vi "3d model.vi"() -> (0 "error out":errorcluster, 1 "Коптер + оси":refnum<vi>, 2 "Вся сцена":refnum<vi>)   [LabVIEW 2013]
uses:
  <vilib>/Utility/miscctls.llb/LV3DPointTypeDef.ctl
  <vilib>/picture/3D Picture Control/Object/Create Object (name).vi
  <vilib>/picture/3D Picture Control/Helpers/Set Light (no reference).vi
  <vilib>/picture/3D Picture Control/NI_3D Picture Control.lvlib
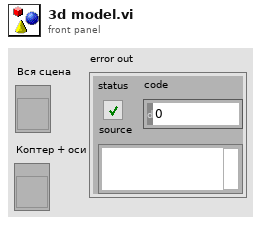
[diagram p1: front panel]
types:
  T1 = cluster{"Red":sgl, "Green":sgl, "Blue":sgl, "Alpha":sgl}
  T2 = typedef "LV3DPointTypeDef.ctl" = cluster{"X":sgl, "Y":sgl, "Z":sgl}
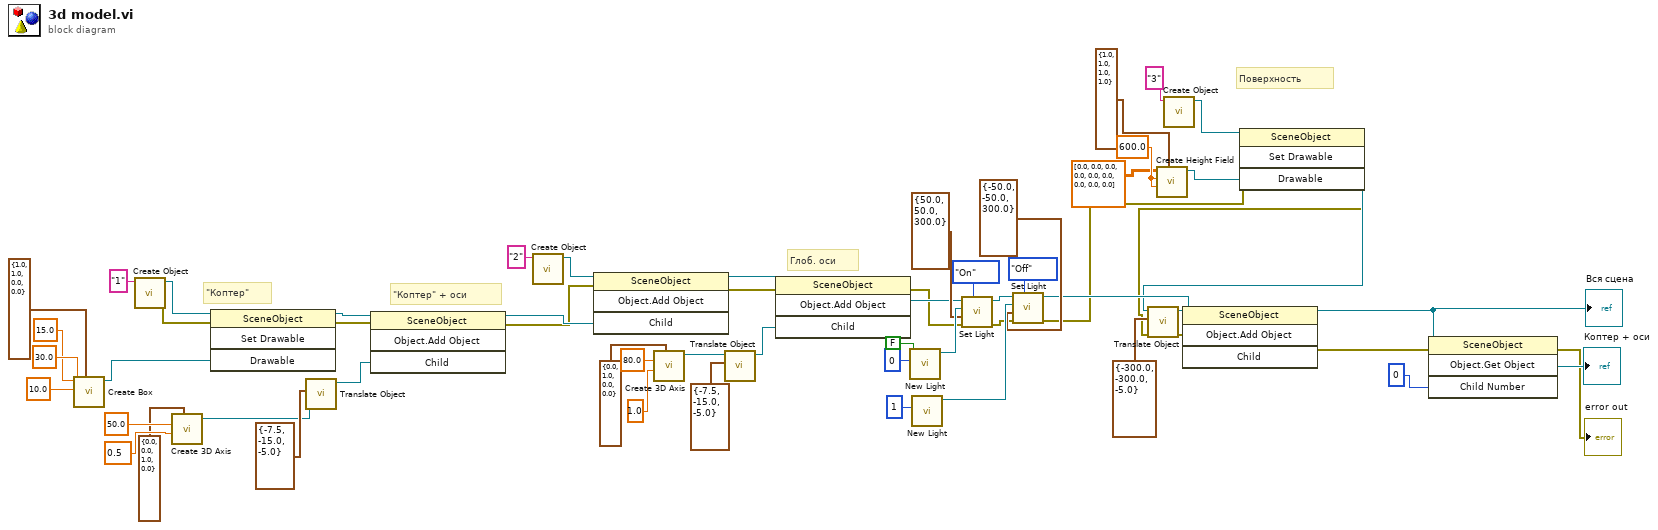
[diagram p0: block diagram]
diagram:
  w44 = sgl 600.0 ("Row Interval")
  # "Глоб. оси"
  # "\"Коптер\" + оси"
  # "\"Коптер\""
  # "Поверхность"
  n1 = call <vilib>:"Create Box.vi"("Color"=T1 {"Red"=1.0, "Green"=1.0, "Blue"=0.0, "Alpha"=0.0}, "Length Z"=sgl 10.0, "Length Y"=sgl 30.0, "Length X"=sgl 15.0) -> ("New Box Refnum"=w15:refnum<vi>)  [unwired: 6 in, 1 out]
  n2 = call-poly <vilib>:"Create Object.vi"("Name"="1") -> ("error out"=w11:errorcluster, "Scene:New Object"=w27:refnum<vi>)  [unwired: 9 in]
  n3 = call <vilib>:"Create 3D Axis.vi"("Color"=T1 {"Red"=0.0, "Green"=0.0, "Blue"=1.0, "Alpha"=0.0}, "Radius"=sgl 0.5, "Length"=sgl 50.0) -> ("New Object Refnum"=w28:refnum<vi>)  [unwired: 7 in, 1 out]
  n4 = invoke class="SceneObject" method="Set Drawable"(reference=w27, error in=w11, "Drawable"=w15) -> (reference out=w33:refnum<vi>, error out=w10:errorcluster)  [unwired: 1 in, 2 out]
  n5 = call <vilib>:"Translate Object.vi"("Translation"=cluster{"X":sgl, "Y":sgl, "Z":sgl} {"X"=-7.5, "Y"=-15.0, "Z"=-5.0}, "Scene.Object In"=w28) -> ("Scene.Object Out"=w34:refnum<vi>)  [unwired: 8 in, 1 out]
  n6 = invoke class="SceneObject" method="Object.Add Object"(reference=w33, error in=w10, "Child"=w34) -> (reference out=w35:refnum<vi>, error out=w9:errorcluster)  [unwired: 1 in, 2 out]
  n7 = call-poly <vilib>:"Create Object.vi"("Name"="2") -> ("Scene:New Object"=w22:refnum<vi>)  [unwired: 9 in, 1 out]
  n8 = invoke class="SceneObject" method="Object.Add Object"(reference=w22, error in=w9, "Child"=w35) -> (reference out=w25:refnum<vi>, error out=w8:errorcluster)  [unwired: 1 in, 2 out]
  n9 = call <vilib>:"Create 3D Axis.vi"("Color"=T1 {"Red"=0.0, "Green"=1.0, "Blue"=0.0, "Alpha"=0.0}, "Radius"=sgl 1.0, "Length"=sgl 80.0) -> ("New Object Refnum"=w20:refnum<vi>)  [unwired: 7 in, 1 out]
  n10 = call <vilib>:"Translate Object.vi"("Translation"=cluster{"X":sgl, "Y":sgl, "Z":sgl} {"X"=-7.5, "Y"=-15.0, "Z"=-5.0}, "Scene.Object In"=w20) -> ("Scene.Object Out"=w26:refnum<vi>)  [unwired: 8 in, 1 out]
  n11 = invoke class="SceneObject" method="Object.Add Object"(reference=w25, error in=w8, "Child"=w26) -> (reference out=w37:refnum<vi>, error out=w7:errorcluster)  [unwired: 1 in, 2 out]
  n12 = call <vilib>:"New Light.vi"("Light Number"=0, "At Infinity"=FALSE) -> ("New Light Refnum"=w50:refnum<vi>)  [unwired: 8 in, 1 out]
  n13 = call <vilib>:"New Light.vi"("Light Number"=1) -> ("New Light Refnum"=w53:refnum<vi>)  [unwired: 9 in, 1 out]
  n14 = call-poly <vilib>:"Set Light.vi"("Light State"=enum16{"Inherit Value", "Off", "On"}."On", "error in (no error)"=w7, "Position"=T2 {"X"=50.0, "Y"=50.0, "Z"=300.0}, "Light Refnum In"=w50, "Scene Object In"=w37) -> ("error out"=w6:errorcluster, "Scene Object Out"=w48:refnum<vi>)  [unwired: 5 in]
  n15 = call-poly <vilib>:"Set Light.vi"("Light State"=enum16{"Inherit Value", "Off", "On"}."Off", "error in (no error)"=w6, "Position"=T2 {"X"=-50.0, "Y"=-50.0, "Z"=300.0}, "Light Refnum In"=w53, "Scene Object In"=w48) -> ("error out"=w5:errorcluster, "Scene Object Out"=w49:refnum<vi>)  [unwired: 5 in]
  n16 = call <vilib>:"Create Height Field.vi"("Color"=T1 {"Red"=1.0, "Green"=1.0, "Blue"=1.0, "Alpha"=1.0}, "Column Interval"=w44, "Row Interval"=w44, "Data"=sgl[][] [[0.0, 0.0, 0.0], [0.0, 0.0, 0.0], [0.0, 0.0, 0.0]]) -> ("New Height Field Refnum"=w42:refnum<vi>)  [unwired: 6 in, 1 out]
  n17 = call-poly <vilib>:"Create Object.vi"("Name"="3") -> ("Scene:New Object"=w41:refnum<vi>)  [unwired: 9 in, 1 out]
  n18 = invoke class="SceneObject" method="Set Drawable"(reference=w41, error in=w5, "Drawable"=w42) -> (reference out=w45:refnum<vi>, error out=w4:errorcluster)  [unwired: 1 in, 2 out]
  n19 = call <vilib>:"Translate Object.vi"("error in (no error)"=w4, "Translation"=cluster{"X":sgl, "Y":sgl, "Z":sgl} {"X"=-300.0, "Y"=-300.0, "Z"=-5.0}, "Scene.Object In"=w45) -> ("error out"=w3:errorcluster, "Scene.Object Out"=w46:refnum<vi>)  [unwired: 7 in]
  n20 = invoke class="SceneObject" method="Object.Add Object"(reference=w49, error in=w3, "Child"=w46) -> (reference out=w59:refnum<vi>, error out=w2:errorcluster)  [unwired: 1 in, 2 out]
  "Вся сцена" <- w59
  n21 = invoke class="SceneObject" method="Object.Get Object"(reference=w59, error in=w2, "Child Number"=0 ("index")) -> (error out=→"error out":errorcluster, "Get Child"=→"Коптер + оси":refnum<vi>)  [unwired: 1 in, 2 out]
